vi "DT Read Encoders.vi"(11 "Reset Encoders":bool) -> ()   [LabVIEW 2017]
uses:
  Robot Global Data.vi
  Common Code/DT Encoder Values.ctl
panel:
  out "Drivetrain Encoder Values":T1
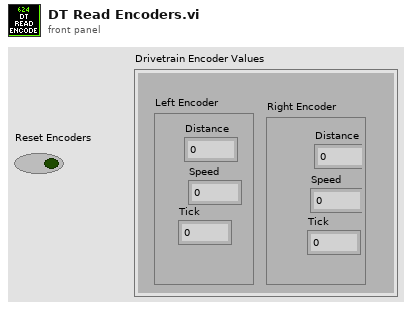
[diagram p1: front panel]
types:
  T1 = cluster{"Left Encoder":cluster{"Distance":dbl, "Speed":dbl, "Tick":dbl}, "Right Encoder":cluster{"Distance":dbl, "Speed":dbl, "Tick":dbl}}
  T2 = typedef "DT Encoder Values.ctl" = cluster{"Left Encoder":cluster{"Distance":dbl, "Speed":dbl, "Tick":dbl}, "Right Encoder":cluster{"Distance":dbl, "Speed":dbl, "Tick":dbl}}
  T3 = typedef "Dashboard Control Data.ctl" = cluster{"Drivetrain Settings Cluster":T4, "Intake Presets":T7, "Elevator Settings Cluster":T8}
  T4 = typedef "Drivetrain Settings Clustr.ctl" = cluster{"Gyro PID Gains":T5, "Drive PID Gains":T5, "Encoder Values":T6, "Drive Tolerance":dbl, "Gyro Tolerance":dbl, "Gyro Output":dbl, "Distance Output":dbl, "Y Power Multiplier":dbl, "Turn Power Multiplier":dbl, "Creep Rate":dbl, "Constant Power":bool, "DT Mode Modifier":enum16{"None, Default", "Cube", "Square"}}
  T5 = typedef "PID Gains Cluster.ctl" = cluster{"Integral Time":dbl, "Proportional Gain":dbl, "Derivative Time":dbl}
  T6 = typedef "Encoder Values.ctl" = cluster{"Distance":dbl, "Speed":dbl, "Tick":dbl}
  T7 = typedef "Intake Presets.ctl" = cluster{"Idle Angle":dbl, "Mid Angle":dbl, "Low Angle":dbl, "Outtake Power":dbl, "Intake Power":dbl, "Unstuck":dbl, "Angle Tolerance":dbl, "Max Angle":dbl, "Max Current":dbl, "Current Trip Time":dbl, "Reset Encoder?":bool, "Encoder Scale":dbl, "PID gains":cluster{"proportional gain (Kc)":dbl, "integral time (Ti, min)":dbl, "derivative time (Td, min)":dbl}, "output range":cluster{"output high":dbl, "output low":dbl}}
  T8 = typedef "Elevator Settings Cluster.ctl" = cluster{"Ground Height":dbl, "Switch Height":dbl, "Scale High Height ":dbl, "Scale Low Height":dbl, "Elevator PID Gains":T9, "Elevator Tolerance":dbl, "Reset Encoders":bool, "Encoder Scale":dbl, "Max Height":dbl, "Mid Height":dbl, "output range":cluster{"output high":dbl, "output low":dbl}}
  T9 = typedef "PID Gains.ctl" = cluster{"proportional gain (Kc)":dbl, "integral time (Ti, min)":dbl, "derivative time (Td, min)":dbl}
  T10 = typedef "WPI_EncoderDevRef.ctl" = cluster{"DevStatus":errorcluster, "EncoderIndex":T11, "CounterIndex":T12, "DistancePerCount":dbl, "Decoding Type":T13}
  T11 = typedef "FPGA_EncoderIdx.ctl" = enum8{"Enc 0", "Enc 1", "Enc 2", "Enc 3", "Enc 4", "Enc 5", "Enc 6", "Enc 7", "Invalid"}
  T12 = typedef "FPGA_CounterCtrSystemIndex.ctl" = enum8{"Ctr 0", "Ctr 1", "Ctr 2", "Ctr 3", "Ctr 4", "Ctr 5", "Ctr 6", "Ctr 7", "Invalid"}
  T13 = typedef "WPI_EncoderType.ctl" = enum16{"1x", "2x", "4x"}
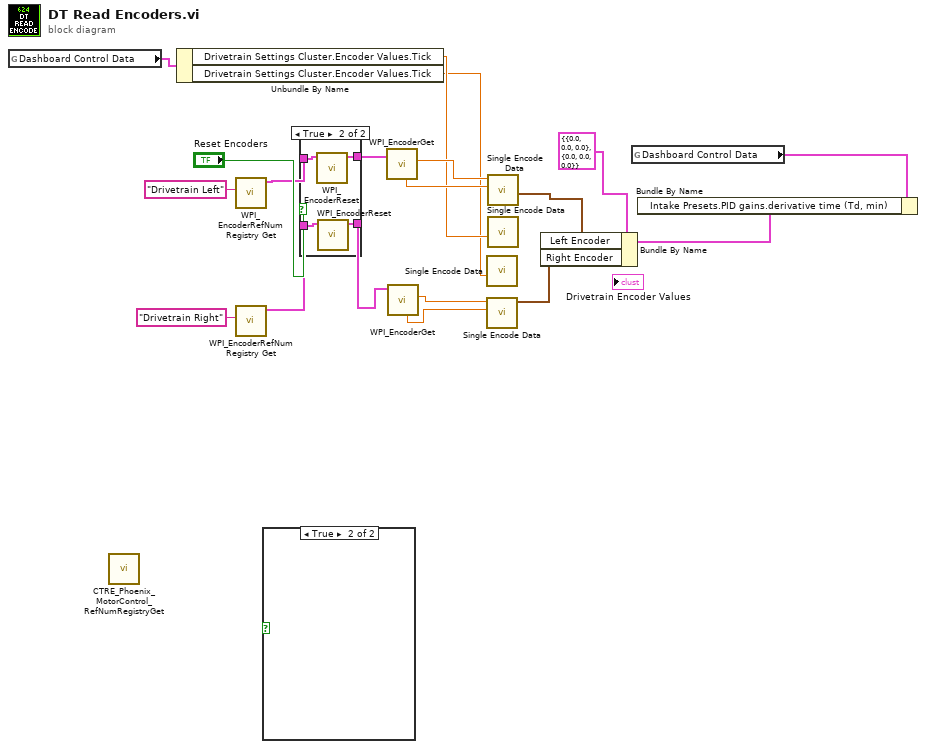
[diagram p0: block diagram]
diagram:
  n1 = global read "Robot Global Data.vi" "Dashboard Control Data"() -> (w3:T3)
  n2 = call "CTRE_Phoenix_MotorControl_RefNumRegistryGet.vi"() -> ()  [unwired: 10 in, 2 out]
  n3 = Unbundle By Name(w3) -> ("Drivetrain Settings Cluster.Encoder Values.Tick"=w2:dbl, "Drivetrain Settings Cluster.Encoder Values.Tick"=w1:dbl)
  n4 = call <vilib>:"WPI_EncoderRefNum Registry Get.vi"("refnum name"="Drivetrain Left") -> ("EncoderDevRef"=w16:T10)  [unwired: 9 in, 1 out]
  n5 = call <vilib>:"WPI_EncoderRefNum Registry Get.vi"("refnum name"="Drivetrain Right") -> ("EncoderDevRef"=w15:T10)  [unwired: 9 in, 1 out]
  n6 = case shown="True" {
    selector: _ -> [_ _]
    frame False {
    }
    frame True {
    }
  }
  n7 = case shown="True" "Reset Encoders" {
    tunnel: w16 -> [w21 w25]
    tunnel: w15 -> [w20 w24]
    tunnel: [w21 w23] -> w14
    tunnel: [w20 w22] -> w13
    frame False {
    }
    frame True {
      n8 = call <vilib>:"WPI_EncoderReset.vi"("EncoderDevRef"=w25) -> ("EncoderDevRef"=w23:T10)  [unwired: 9 in, 1 out]
      n9 = call <vilib>:"WPI_EncoderReset.vi"("EncoderDevRef"=w24) -> ("EncoderDevRef"=w22:T10)  [unwired: 9 in, 1 out]
    }
  }
  n10 = call <vilib>:"WPI_EncoderGet.vi"("EncoderDevRef"=w14) -> ("Distance"=w9:dbl, "Rate"=w10:dbl)  [unwired: 5 in, 4 out]
  n11 = call <vilib>:"WPI_EncoderGet.vi"("EncoderDevRef"=w13) -> ("Distance"=w11:dbl, "Rate"=w12:dbl)  [unwired: 5 in, 4 out]
  n12 = call "Single Encode Data.vi"("Tick Constant"=w1) -> ()  [unwired: 10 in, 1 out]
  n13 = call "Single Encode Data.vi"("Rate"=w12, "Distance"=w11) -> ("Encoder Values"=w5:T6)  [unwired: 9 in]
  n14 = call "Single Encode Data.vi"("Rate"=w10, "Distance"=w9) -> ("Encoder Values"=w6:T6)  [unwired: 9 in]
  n15 = call "Single Encode Data.vi"("Tick Constant"=w2) -> ()  [unwired: 10 in, 1 out]
  n16 = Bundle By Name(cluster=T2 {"Left Encoder"={"Distance"=0.0, "Speed"=0.0, "Tick"=0.0}, "Right Encoder"={"Distance"=0.0, "Speed"=0.0, "Tick"=0.0}} ("Drivetrain Encoder Values"), "Left Encoder"=w6, "Right Encoder"=w5) -> (w8:T2)
  n17 = global read "Robot Global Data.vi" "Dashboard Control Data"() -> (w4:T3)
  n18 = Bundle By Name(cluster=w4, "Intake Presets.PID gains.derivative time (Td, min)"=w8) -> ()  [unwired: 1 out]
